vi "Device Reset.vi"(8 "error in (no error)":errorcluster) -> (0 "error out":errorcluster, 3 "Reset OK?":bool)   [LabVIEW 2015, in "ST-Link.lvlib"]
doc: "复位芯片。\n\n[Reset OK?]: 返回复位状态；"
uses:
  ST-Link.lvlib
panel:
  out "standard output":string
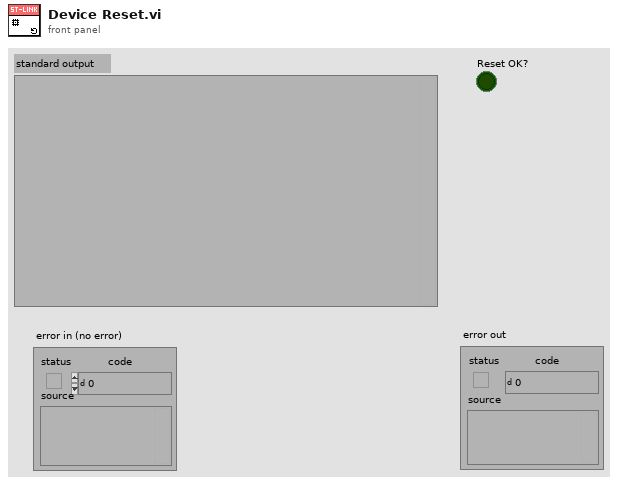
[diagram p1: front panel]
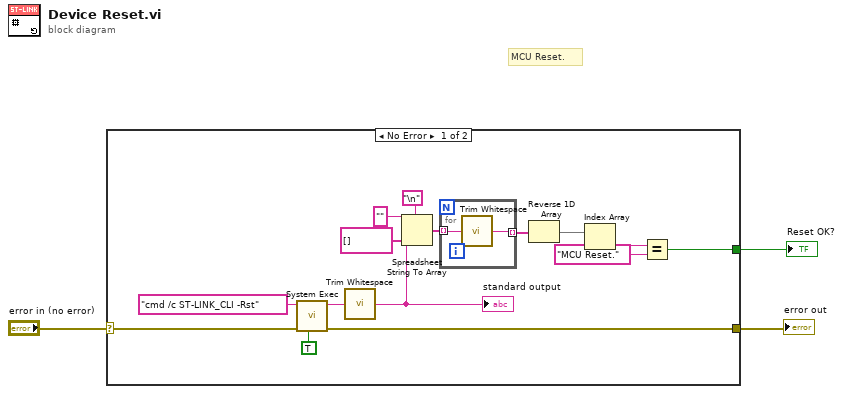
[diagram p0: block diagram]
diagram:
  # "MCU Reset."
  n1 = case shown="No Error" "error in (no error)" {
    selector: "error in (no error)" -> [w16 w21]
    tunnel: [w15 w21] -> w2
    tunnel: [w4 _] -> w1
    frame No Error {
      n2 = call <vilib>:"System Exec.vi"("run minimized? (F)"=TRUE, "error in (no error)"=w16, "command line"="cmd /c ST-LINK_CLI -Rst") -> ("error out"=w15:errorcluster, "standard output"=w14:string)  [unwired: 5 in, 2 out]
      n3 = call <vilib>:"Trim Whitespace.vi"("string"=w14) -> ("trimmed string"=w8:string)  [unwired: 1 in]
      "standard output" <- w8
      n4 = Spreadsheet String To Array(delimiter (Tab)="\n", format string="", spreadsheet string=w8, array type (2D Dbl)=string[] []) -> (array=w10:string[])
      n5 = for {
        tunnel: w10 -> [w20] mode=indexing
        tunnel: [w19] -> w9 mode=indexing
        n6 = call <vilib>:"Trim Whitespace.vi"("string"=w20) -> ("trimmed string"=w19:string)  [unwired: 1 in]
      }
      n7 = Reverse 1D Array(array=w9) -> (reversed array=w7:string[])
      n8 = Index Array(array=w7) -> (element=w6:string)  [unwired: 1 in]
      n9 = Equal?(x=w6, y="MCU Reset.") -> (x = y?=w4:bool)
    }
    frame Error {
    }
  }
  "error out" <- w2
  "Reset OK?" <- w1
